vi "InitializeDAQs.vi"(10 "Experiment State":T1={"Send Trigger 3"=FALSE, "error"={"status"=FALSE, "code"=0, "source"=""}, "Digitizer DAQmx Tasks"={"TaskArray"=[]}, "Digitizer Settings"={"6133 Digitizer Channels"=[], "Global Edge Type"=10280, "Total Samples"=[], "Pre-Trigger Samples"=[], "Sample Rate"=[], "Trigger Sources"=[], "Voltage Ranges"=[], "Channel Names"=[], "Active"=[], "Samples to remove"=[], "Start Time"=[], "End Time"=[]}, "Timing Card 2 Fast Outputs"=[{"Delay (s)"=2.559999942779541, "Pulse width (s)"=0.009999999776482582, "Active"=TRUE, "Channel Name"="Fiber 8", "counter"="PXI1Slot8/ctr7"}], "Synchronization Card Settings"={"Position"="PXI1Slot2", "source terminal"="GlobalSoftwareTrigger"}, "Digitizer Data"=[], "Next Shot#"="0", "Timing Card 1 Settings"={"Slot 8 Trigger Source"="", "Clock Source"="", "Trigger Channel Tasks"=[]}, "Timing Card 2 Settings"={"Clock Source"="", "Slot 9 Trigger Source"="", "Trigger Channel Tasks"=[]}, "Timing Card 1 Fast Outputs"=[{"Delay (s)"=2.559999942779541, "Pulse width (s)"=0.009999999776482582, "Active"=TRUE, "Channel Name"="Fiber 8", "counter"="PXI1Slot8/ctr7"}], "System Message"="", "User Shot Notes"=""} {"Timing Card 1 Fast Outputs"."Pulse width (s)" format="%.3p"; "Timing Card 1 Fast Outputs"."Delay (s)" format="%.3p"; "Timing Card 2 Fast Outputs"."Pulse width (s)" format="%.3p"; "Timing Card 2 Fast Outputs"."Delay (s)" format="%.3p"; "Digitizer Settings"."Sample Rate" format="%#_3p"; "Digitizer Settings"."Global Edge Type" items=["Rising"=10280, "Falling"=10171]}) -> (2 "Experiment State":T1={"Send Trigger 3"=FALSE, "error"={"status"=FALSE, "code"=0, "source"=""}, "Digitizer DAQmx Tasks"={"TaskArray"=[]}, "Digitizer Settings"={"6133 Digitizer Channels"=[], "Global Edge Type"=10280, "Total Samples"=[], "Pre-Trigger Samples"=[], "Sample Rate"=[], "Trigger Sources"=[], "Voltage Ranges"=[], "Channel Names"=[], "Active"=[], "Samples to remove"=[], "Start Time"=[], "End Time"=[]}, "Timing Card 2 Fast Outputs"=[{"Delay (s)"=2.559999942779541, "Pulse width (s)"=0.009999999776482582, "Active"=TRUE, "Channel Name"="Fiber 8", "counter"="PXI1Slot8/ctr7"}], "Synchronization Card Settings"={"Position"="PXI1Slot2", "source terminal"="GlobalSoftwareTrigger"}, "Digitizer Data"=[], "Next Shot#"="0", "Timing Card 1 Settings"={"Slot 8 Trigger Source"="", "Clock Source"="", "Trigger Channel Tasks"=[]}, "Timing Card 2 Settings"={"Clock Source"="", "Slot 9 Trigger Source"="", "Trigger Channel Tasks"=[]}, "Timing Card 1 Fast Outputs"=[{"Delay (s)"=2.559999942779541, "Pulse width (s)"=0.009999999776482582, "Active"=TRUE, "Channel Name"="Fiber 8", "counter"="PXI1Slot8/ctr7"}], "System Message"="", "User Shot Notes"=""} {"Timing Card 1 Fast Outputs"."Pulse width (s)" format="%.3p"; "Timing Card 1 Fast Outputs"."Delay (s)" format="%.3p"; "Timing Card 2 Fast Outputs"."Pulse width (s)" format="%.3p"; "Timing Card 2 Fast Outputs"."Delay (s)" format="%.3p"; "Digitizer Settings"."Sample Rate" format="%#_3p"; "Digitizer Settings"."Global Edge Type" items=["Rising"=10280, "Falling"=10171]})   [LabVIEW 2013]
uses:
  Controls/ExperimentStateCluster.ctl
  <vilib>/DAQmx/configure/timing.llb/DAQmx Timing (Sample Clock).vi
  <vilib>/DAQmx/configure/trigger.llb/DAQmx Reference Trigger (Digital Edge).vi
  <vilib>/DAQmx/create/channels.llb/DAQmx Create Channel (AI-Voltage-Basic).vi
panel:
  # "Channel Settings"
  # "Card Wide Settings"
  # "Channel Settings"
  # "Card Wide Settings"
types:
  T1 = typedef "ExperimentStateCluster.ctl" = cluster{"Send Trigger 3":bool, "error":errorcluster, "Digitizer DAQmx Tasks":cluster{"TaskArray":refnum<k21>[]}, "Digitizer Settings":cluster{"6133 Digitizer Channels":tag[][], "Global Edge Type":i32, "Total Samples":i32[], "Pre-Trigger Samples":u32[], "Sample Rate":dbl[], "Trigger Sources":tag[], "Voltage Ranges":dbl[][], "Channel Names":string[][], "Active":bool[][], "Samples to remove":u32[], "Start Time":dbl[], "End Time":dbl[]}, "Timing Card 2 Fast Outputs":cluster{"Delay (s)":dbl, "Pulse width (s)":dbl, "Active":bool, "Channel Name":string, "counter":tag}[], "Synchronization Card Settings":cluster{"Position":refnum<k15>, "source terminal":string}, "Digitizer Data":waveform(dbl)[][], "Next Shot#":string, "Timing Card 1 Settings":cluster{"Slot 8 Trigger Source":tag, "Clock Source":tag, "Trigger Channel Tasks":refnum<k21>[]}, "Timing Card 2 Settings":cluster{"Clock Source":tag, "Slot 9 Trigger Source":tag, "Trigger Channel Tasks":refnum<k21>[]}, "Timing Card 1 Fast Outputs":cluster{"Delay (s)":dbl, "Pulse width (s)":dbl, "Active":bool, "Channel Name":string, "counter":tag}[], "System Message":string, "User Shot Notes":string}
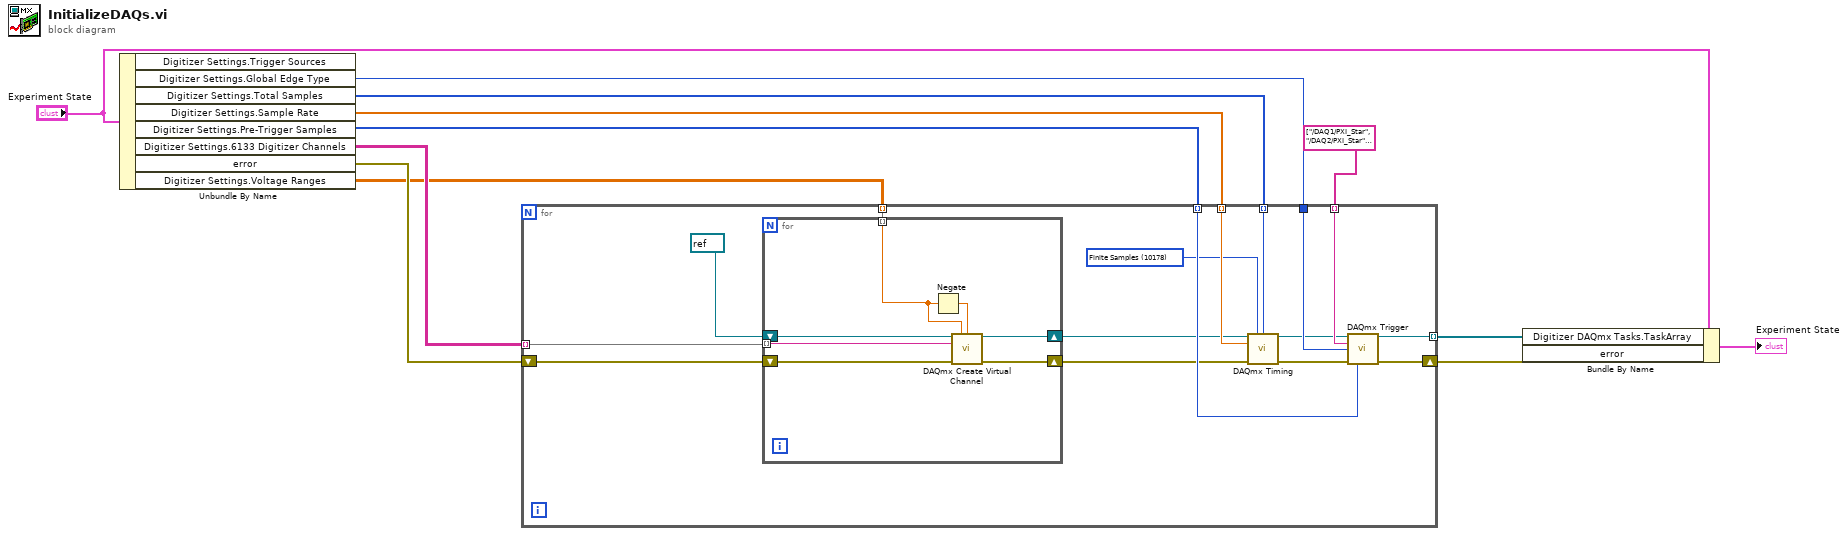
[diagram p0: block diagram]
diagram:
  n1 = Unbundle By Name("Experiment State") -> ("Digitizer Settings.Global Edge Type"=w9:i32, "Digitizer Settings.Total Samples"=w6:i32[], "Digitizer Settings.Sample Rate"=w5:dbl[], "Digitizer Settings.Pre-Trigger Samples"=w4:u32[], "Digitizer Settings.6133 Digitizer Channels"=w8:tag[][], "error"=w7:errorcluster, "Digitizer Settings.Voltage Ranges"=w2:dbl[][])  [unwired: 1 out]
  n2 = for {
    tunnel: tag[] ["/DAQ1/PXI_Star", "/DAQ2/PXI_Star", "/DAQ3/PXI_Star"] ("Trigger Sources") -> [w27] mode=indexing
    tunnel: w9 -> [w26]
    tunnel: w6 -> [w25] mode=indexing
    tunnel: w5 -> [w24] mode=indexing
    tunnel: w4 -> [w23] mode=indexing
    tunnel: w8 -> [w22] mode=indexing
    tunnel: [w19] -> w3 mode=indexing
    shift-right: [w28] -> w10
    shift-left: w7 -> [w21]
    tunnel: w2 -> [w13] mode=indexing
    w16 = 10178 items=["Finite Samples"=10178, "Continuous Samples"=10123, "Hardware Timed Single Point"=12522] ("sample mode")
    n3 = for {
      tunnel: w22 -> [w35] mode=indexing
      shift-right: [w32] -> w18
      shift-left: refnum<k21> refnum ("task out") -> [w33]
      shift-right: [w31] -> w17
      shift-left: w21 -> [w34]
      tunnel: w13 -> [w29] mode=indexing
      n4 = Negate(x=w29) -> (-x=w30:dbl)
      n5 = call-poly <vilib>:"DAQmx Create Virtual Channel.vi"("task in"=w33, "maximum value"=w29, "minimum value"=w30, "physical channels"=w35, "error in"=w34) -> ("task out"=w32:refnum<k21>, "error out"=w31:errorcluster)  [unwired: 4 in, 5 out]
    }
    n6 = call-poly <vilib>:"DAQmx Timing.vi"("task/channels in"=w18, "sample mode"=w16, "samples per channel"=w25, "rate"=w24, "error in"=w17) -> ("task out"=w15:refnum<k21>, "error out"=w14:errorcluster)  [unwired: 2 in, 7 out]
    n7 = call-poly <vilib>:"DAQmx Trigger.vi"("task/channels in"=w15, "source"=w27, "edge"=w26, "error in"=w14, "pretrigger samples per channel"=w23) -> ("task out"=w19:refnum<k21>, "error out"=w28:errorcluster)  [unwired: 9 out]
  }
  n8 = Bundle By Name(cluster="Experiment State", "Digitizer DAQmx Tasks.TaskArray"=w3, "error"=w10) -> (→"Experiment State":T1)
